vi "NI知识库智能助手.vi"() -> ()   [LabVIEW 2023]
uses:
  RAG_LV_API/LabVIEW RAG.lvlib
  labview-local-model/LabVIEW LLM.lvlib
  labview-ai-share/LabVIEW AI Base.lvlib
panel:
  in  "Tab Control":enum32{"Standard", "Advanced"}(tab)
  in  "Question:":string(combo)="NI 9230有多少个模拟输入？"
  in  "Knowledge Base Name":string="NI-cDAQ"
  out "Answer":string
  out "error out":errorcluster
  in  "OpenAI-Compatible LLM URL":string(combo)="https://openrouter.ai/api/v1"
  in  "LLM Model Name":string(combo)="qwen/qwq-32b:free"
  in  "API Key":string(combo)="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"
  in  "K":u32=5
  in  "Temperature":dbl=0.2
  in  "System Prompt":string="Note that when users ask questions about NI hardware (like cDAQ), cDAQ-9219 is the same hardware as NI-9219 or \"NI 9219\" or \"NI-9219\"."
  in  "reasoning":T1={"effort"=enum."low", "exclude"=FALSE}
  in  "Python venv path":path=path "C:/dev/gaoruhao/labview-ai"
  in  "Python version":string="3.10"
  # "NI知识库智能助手"
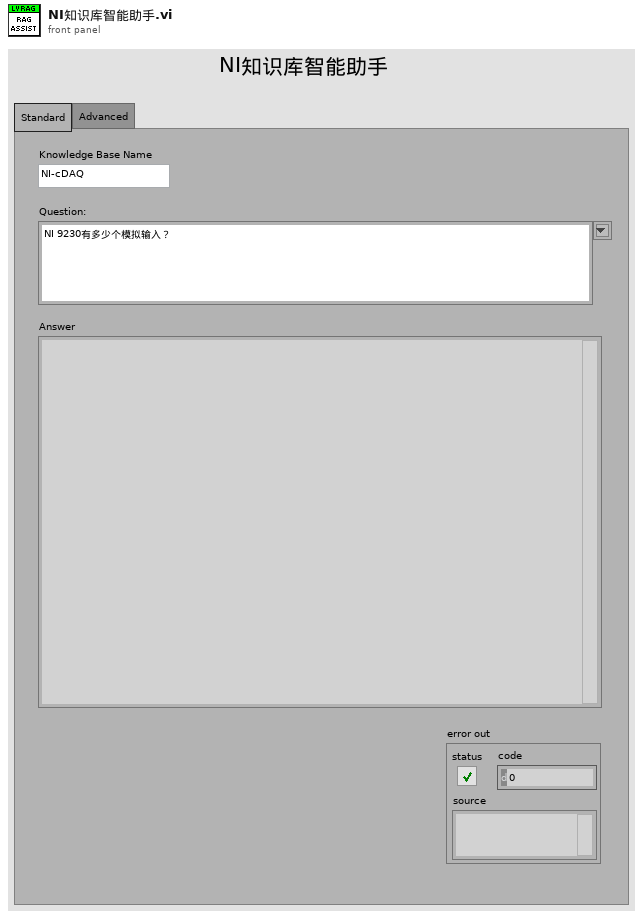
[diagram p1: front panel]
types:
  T1 = cluster{"effort":enum16{"high", "medium", "low"}, "exclude":bool}
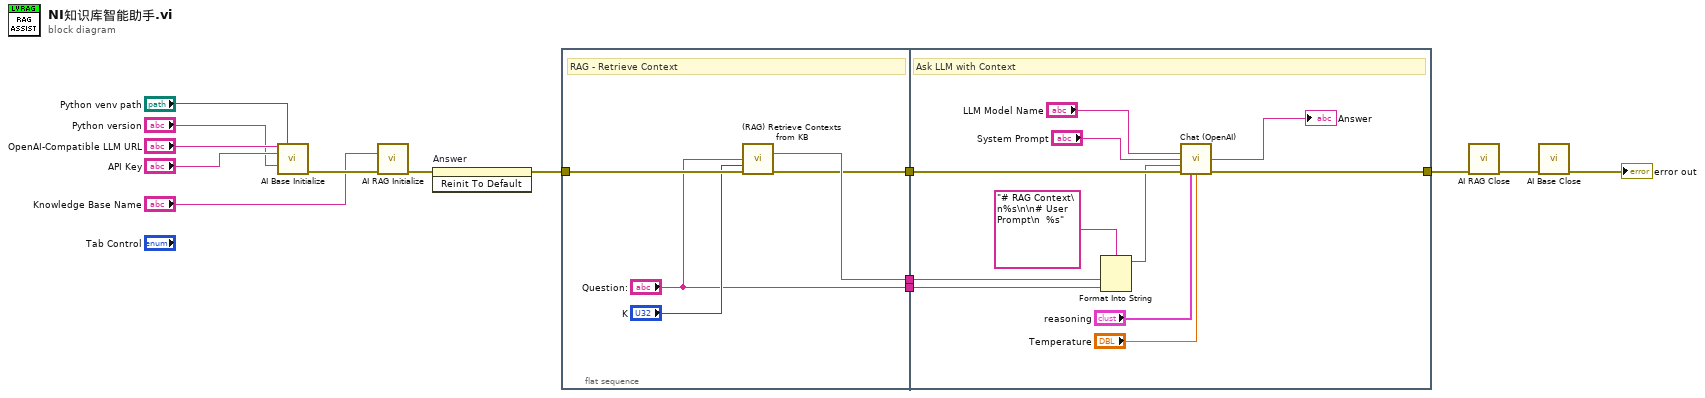
[diagram p0: block diagram]
diagram:
  n1 = call "AI Base Initialize.vi"("OpenAI API URL"="OpenAI-Compatible LLM URL", "Python venv path"="Python venv path", "API Key"="API Key", "Python version"="Python version") -> ("error out"=w5:errorcluster)  [unwired: 9 in, 2 out]
  n2 = call "AI RAG Initialize.vi"("Knowledge Base Name"="Knowledge Base Name", "error in (no error)"=w5) -> ("error out"=w3:errorcluster)  [unwired: 13 in]
  n3 = invoke on="Answer" class="Str" method="Reinit To Default"(error in=w3) -> (error out=w4:errorcluster)  [unwired: 2 in, 2 out]
  n4 = flat-sequence {
    tunnel: [w17] -> w9
    tunnel: [w18] -> w8
    tunnel: ["Question:"] -> w7
    tunnel: w4 -> [w19]
    tunnel: [w29] -> w13
    tunnel: w9 -> [w30]
    tunnel: w8 -> [w27]
    tunnel: w7 -> [w25]
    frame #0 {
      # "RAG - Retrieve Context"
      n5 = call "(RAG) Retrieve Contexts from KB.vi"("RAG Query"="Question:", "K"="K", "error in"=w19) -> ("Retrieved Contexts"=w18:string, "error out"=w17:errorcluster)  [unwired: 10 in, 1 out]
    }
    frame #1 {
      # "Ask LLM with Context"
      n6 = Format Into String(format string="# RAG Context\n%s\n\n# User Prompt\n  %s", w27, w25) -> (resulting string=w23:string)  [unwired: 2 in, 1 out]
      n7 = call "Chat (OpenAI).vi"("LLM Model Name"="LLM Model Name", "System Prompt"="System Prompt", "User Prompt"=w23, "error in"=w30, "reasoning"="reasoning", "Temperature"="Temperature") -> ("Answer content"=→"Answer":string, "error out"=w29:errorcluster)  [unwired: 5 in, 3 out]
    }
  }
  n8 = call "AI RAG Close.vi"("error in"=w13) -> ("error out"=w2:errorcluster)  [unwired: 10 in]
  n9 = call "AI Base Close.vi"("error in"=w2) -> ("error out"=→"error out":errorcluster)  [unwired: 10 in]
